vi "VG-createUserEvents.vi"(8 "error in (no error)":errorcluster, 11 "VG-VNA_GUI in":refnum<class "VG-VNA_GUI.lvclass">) -> (0 "error out":errorcluster, 3 "VG-VNA_GUI out":refnum<class "VG-VNA_GUI.lvclass">)   [LabVIEW 2020, in "VG-VNA_GUI.lvlib" / "VG-VNA_GUI.lvclass"]
uses:
  VG-VNA_GUI.lvclass
  VG-graph_data.ctl
  VG-VNA_GUI.lvclass/VG-VNA_GUI.ctl
  data_handler/VDH-VNA_data_handler/VDH-VNA_data_handler/VDH-calibration_status.ctl
  data_handler/VDH-VNA_data_handler/VDH-VNA_data_handler/VDH-SOLT_calib_Status.ctl
  data_handler/VDH-VNA_data_handler/VDH-VNA_data_handler/VDH-Calibration_prosess.ctl
  data_handler/VDH-VNA_data_handler/VDH-VNA_data_handler/VDH-Calibration_enum.ctl
  hardware_manager/VHM-VNA_Hardware_Manager/VHM-VNA_Hardware_Manager/VHM-connection_status.ctl
  data_handler/VDH-VNA_data_handler/VDH-VNA_data_handler/VDH-VNA_data_handler.lvclass
  hardware_manager/VHM-VNA_Hardware_Manager/VHM-VNA_Hardware_Manager/VHM-VNA_Hardware_Manager.lvclass
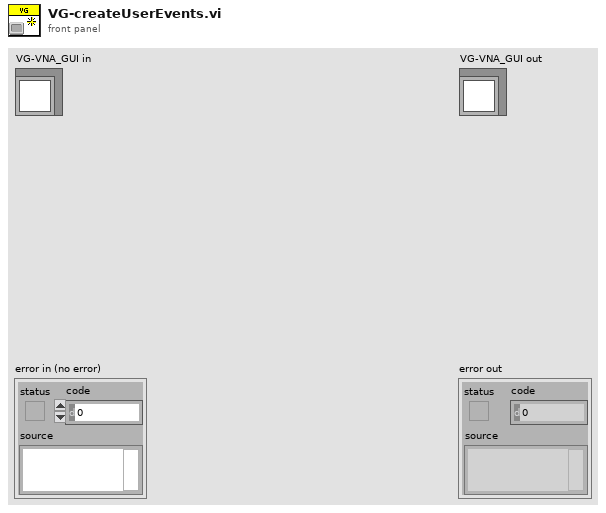
[diagram p1: front panel]
types:
  T1 = typedef "VG-VNA_GUI.lvlib/VG-VNA_GUI.lvclass/VG-graph_data.ctl" = cluster{u64[], dbl[]}[]
  T2 = typedef "VHM-VNA_Hardware_Manager.lvlib/VHM-VNA_Hardware_Manager.lvclass/VHM-connection_status.ctl" = cluster{"Connected?":bool, "Status":string}
  T3 = typedef "VDH-VNA_data_handler.lvlib/VDH-VNA_data_handler.lvclass/VDH-calibration_status.ctl" = cluster{"Calib Status":T4, "Calibrated?":bool, "Permativity?":bool, "Progress":T5}
  T4 = typedef "VDH-VNA_data_handler.lvlib/VDH-VNA_data_handler.lvclass/VDH-SOLT_calib_Status.ctl" = cluster{"Short":bool, "Open":bool, "Load":bool, "Through":bool}
  T5 = typedef "VDH-VNA_data_handler.lvlib/VDH-VNA_data_handler.lvclass/VDH-Calibration_prosess.ctl" = cluster{"Progress":bool, "current":T6, "samples to get":u8}
  T6 = typedef "VDH-VNA_data_handler.lvlib/VDH-VNA_data_handler.lvclass/VDH-Calibration_enum.ctl" = enum16{"Non", "Short", "Open", "Load", "Through", "Permativity"}
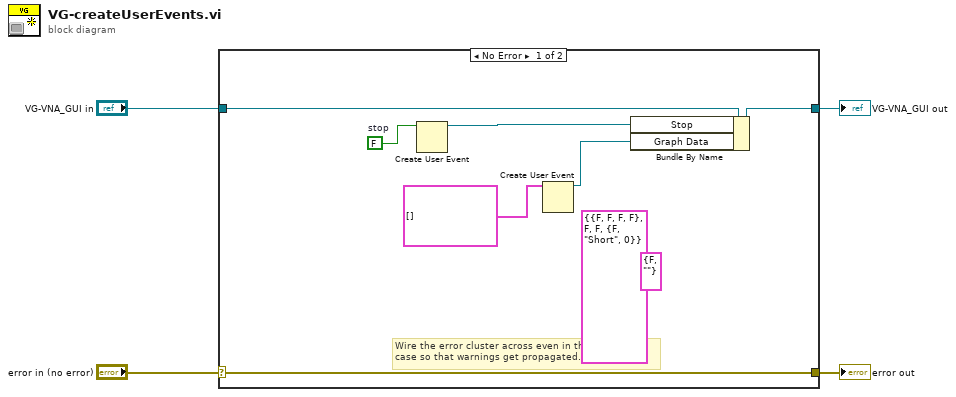
[diagram p0: block diagram]
diagram:
  n1 = case shown="No Error" "error in (no error)" {
    selector: "error in (no error)" -> [w10 w13]
    tunnel: [w10 w13] -> w3
    tunnel: [w7 w12] -> w1
    tunnel: "VG-VNA_GUI in" -> [w11 w12]
    frame No Error {
      (unwired) T2 {"Connected?"=FALSE, "Status"=""} ("connection status")
      (unwired) T3 {"Calib Status"={"Short"=FALSE, "Open"=FALSE, "Load"=FALSE, "Through"=FALSE}, "Calibrated?"=FALSE, "Permativity?"=FALSE, "Progress"={"Progress"=FALSE, "current"=enum."Short", "samples to get"=0}} ("Calibration Status")
      w9 = FALSE  # stop
      # "Wire the error cluster across even in the \"No Error\"\ncase so that warnings get propagated."
      n2 = Create User Event(user event datatype=w9) -> (user event=w6:refnum<user-event>)  [unwired: 1 in, 1 out]
      n3 = Create User Event(user event datatype=T1 [] ("Graph Data")) -> (user event=w5:refnum<user-event>)  [unwired: 1 in, 1 out]
      n4 = Bundle By Name(cluster=w11, "Stop"=w6, "Graph Data"=w5) -> (w7:refnum<class "VG-VNA_GUI.lvclass">)
    }
    frame Error {
    }
  }
  "error out" <- w3
  "VG-VNA_GUI out" <- w1
